vi "Stage 3.5 Placing init and close into subVIs.vi"() -> ()   [LabVIEW 2020]
uses:
  HRM-User_events.ctl
panel:
  out "Process Error":errorcluster
  out "error out":errorcluster
  out "error out Hardware":errorcluster
  in  "Addition signal to remove (0) [s]":dbl
  out "Pulse":dbl
  out "Filtered":waveform(dbl)(graph)
  in  "Samples size (10) [s]":i32=10
  out "unfiltered wf":waveform(dbl)(graph)
  in  "Stop":bool
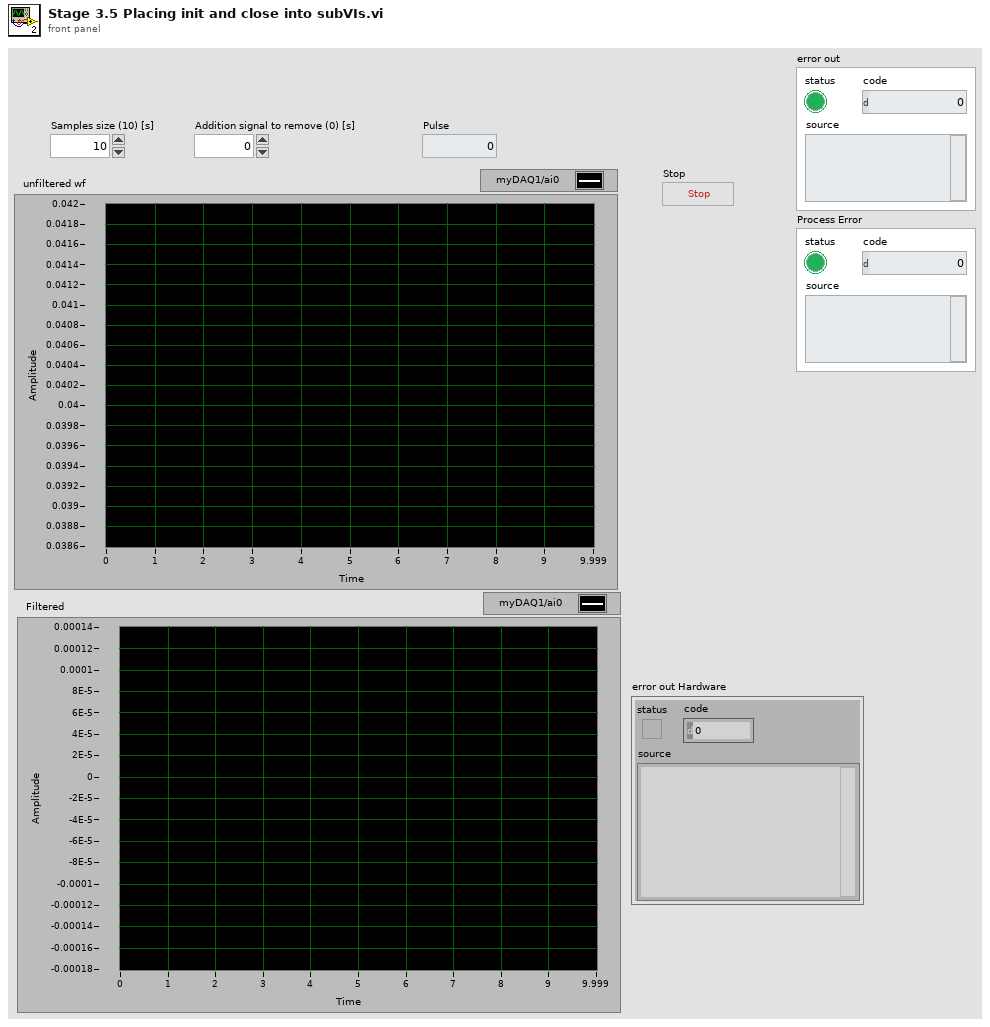
[diagram p1: front panel]
types:
  T1 = typedef "HRM-User_events.ctl" = cluster{"Signal to remove":refnum<user-event>, "Sample size":refnum<user-event>, "Filtered wf":refnum<user-event>, "Unfiltered wf":refnum<user-event>, "Raw wf":refnum<user-event>, "Pulse":refnum<user-event>, "stop":refnum<user-event>}
  T2 = typedef "HRM-init_cluster.ctl" = cluster{"User events":T1}
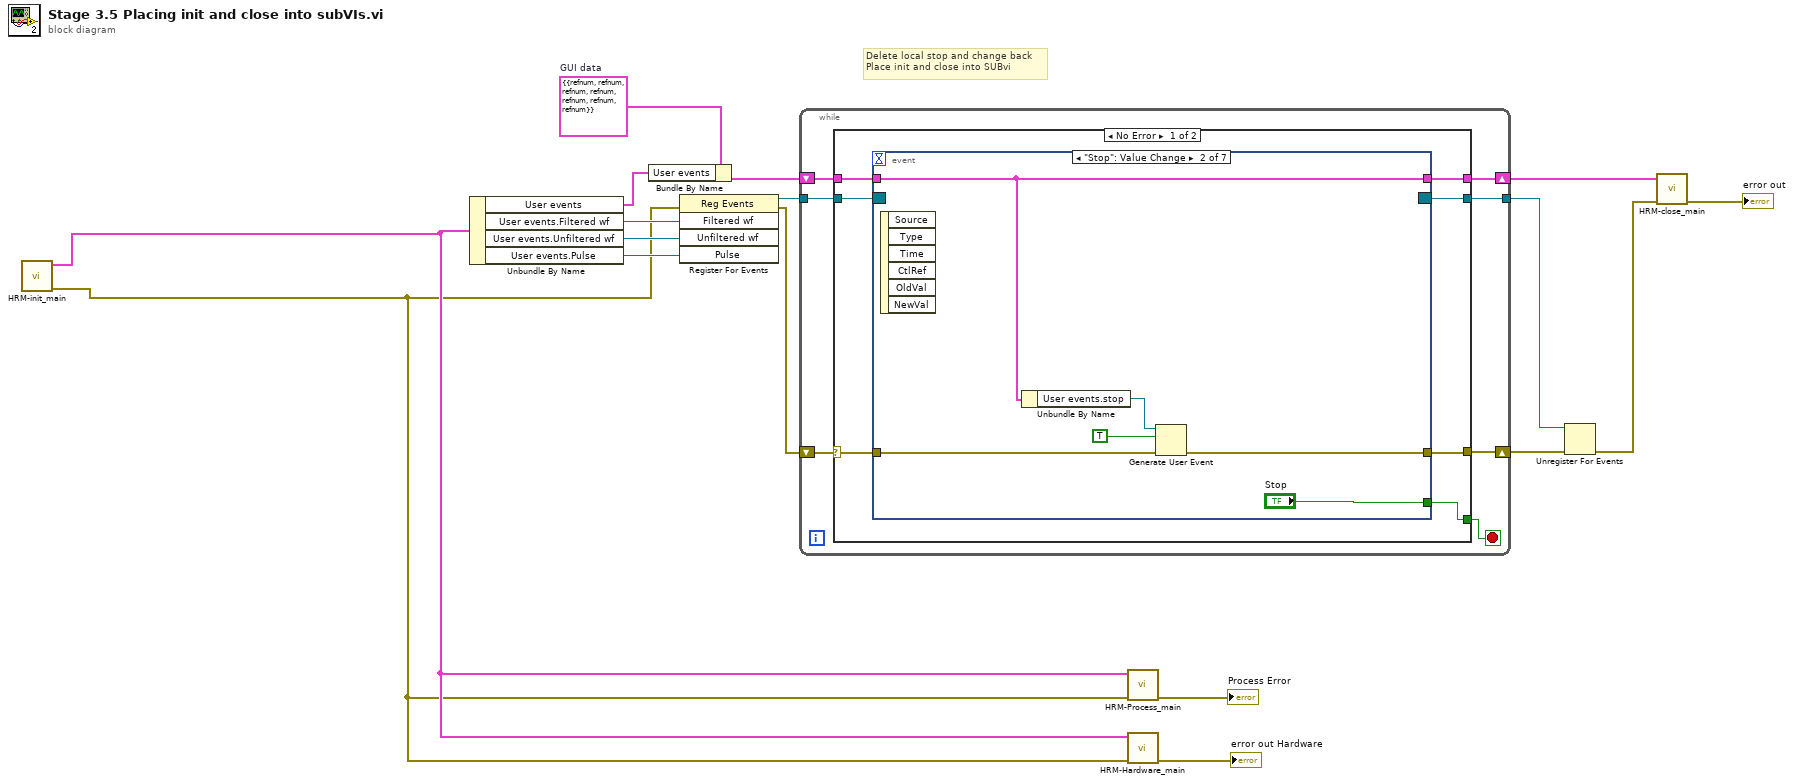
[diagram p0: block diagram]
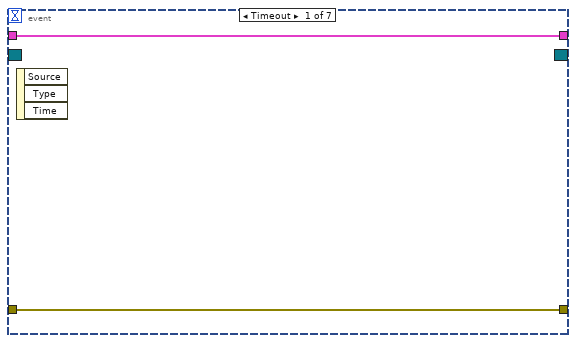
[diagram p2: hidden frame]
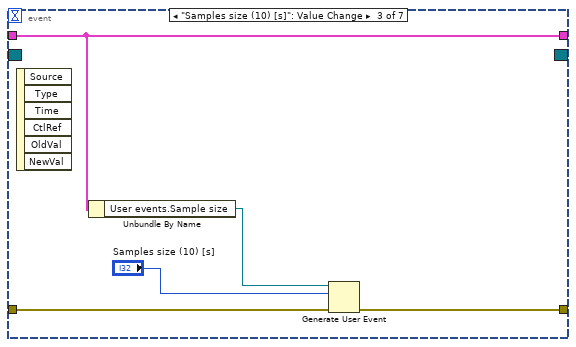
[diagram p3: hidden frame]
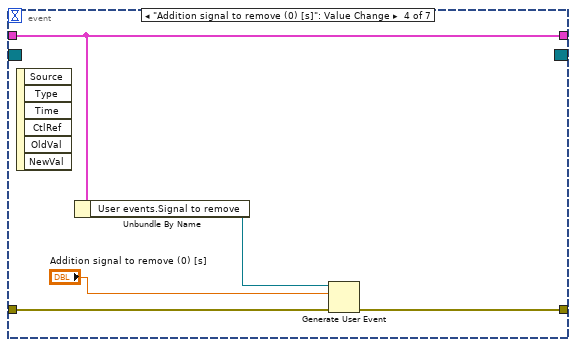
[diagram p4: hidden frame]
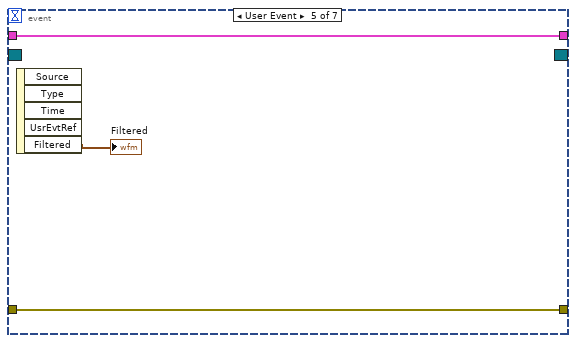
[diagram p5: hidden frame]
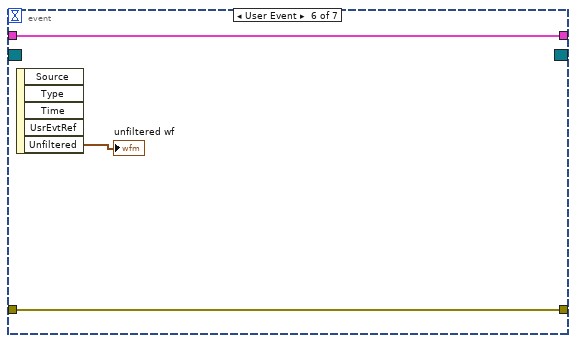
[diagram p6: hidden frame]
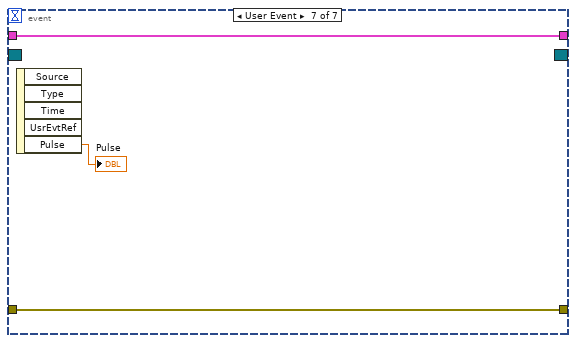
[diagram p7: hidden frame]
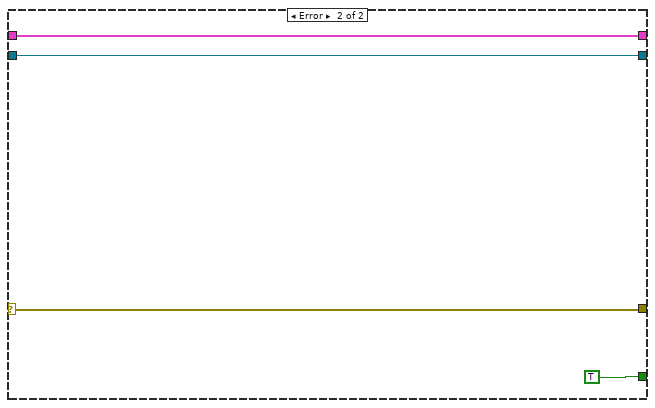
[diagram p8: hidden frame]
diagram:
  w16 = cluster{"User events":T1} {"User events"={"Signal to remove"=refnum, "Sample size"=refnum, "Filtered wf"=refnum, "Unfiltered wf"=refnum, "Raw wf"=refnum, "Pulse"=refnum, "stop"=refnum}}  # GUI data
  # "Delete local stop and change back\nPlace init and close into SUBvi"
  n1 = call "HRM-init_main.vi"() -> ("error out"=w1:errorcluster, "Init cluster"=w3:T2)  [unwired: 10 in]
  n2 = Unbundle By Name(w3) -> ("User events"=w8:T1, "User events.Filtered wf"=w7:refnum<user-event>, "User events.Unfiltered wf"=w6:refnum<user-event>, "User events.Pulse"=w5:refnum<user-event>)
  n3 = Bundle By Name(cluster=w16, "User events"=w8) -> (w9:cluster{"User events":T1})
  n4 = register-events(error in=w1, w7, w6, w5) -> (reference out=w17:refnum<event-registration>, error out=w15:errorcluster)  [unwired: 1 in]
  n5 = while {
    tunnel: w17 -> [w24]
    shift-right: [w20] -> w13
    shift-left: w15 -> [w21]
    shift-right: [w19] -> w12
    shift-left: w9 -> [w23]
    tunnel: [w18] -> w14
    stop <- w22 stop-if-true
    n6 = case shown="No Error" w21 {
      selector: w21 -> [w28 w61]
      tunnel: [w29 TRUE ("Stop")] -> w22
      tunnel: [w27 w61] -> w20
      tunnel: w24 -> [w31 w59]
      tunnel: w23 -> [w30 w60]
      tunnel: [w26 w60] -> w19
      tunnel: [w25 w59] -> w18
      frame No Error {
        n7 = event shown="[1] \"Stop\": Value Change" {
          selector: w31 -> [_ _ _ _ _ _ _]
          dyn-events: [_ _ _ _ _ _ _] -> w25
          timeout: _ -> [_ _ _ _ _ _ _]
          tunnel: w30 -> [w33 w38 w42 w47 w51 w54 w57]
          tunnel: [_ "Stop" _ _ _ _ _] -> w29
          tunnel: [w32 w35 w43 w48 w52 w55 w58] -> w27
          tunnel: w28 -> [w32 w36 w44 w49 w52 w55 w58]
          tunnel: [w33 w38 w42 w47 w51 w54 w57] -> w26
          event Timeout {
            n8 = event-data() -> ()  [unwired: 1 in, 3 out]
          }
          event "Stop": Value Change {
            n9 = event-data() -> ()  [unwired: 1 in, 6 out]
            n10 = Unbundle By Name(w38) -> ("User events.stop"=w37:refnum<user-event>)
            n11 = Generate User Event(user event=w37, event data cluster=TRUE ("event data"), error in=w36) -> (error out=w35:errorcluster)  [unwired: 1 in, 1 out]
          }
          event "Samples size (10) [s]": Value Change {
            n12 = event-data() -> ()  [unwired: 1 in, 6 out]
            n13 = Unbundle By Name(w42) -> ("User events.Sample size"=w41:refnum<user-event>)
            n14 = Generate User Event(user event=w41, event data cluster="Samples size (10) [s]", error in=w44) -> (error out=w43:errorcluster)  [unwired: 1 in, 1 out]
          }
          event "Addition signal to remove (0) [s]": Value Change {
            n15 = event-data() -> ()  [unwired: 1 in, 6 out]
            n16 = Unbundle By Name(w47) -> ("User events.Signal to remove"=w46:refnum<user-event>)
            n17 = Generate User Event(user event=w46, event data cluster="Addition signal to remove (0) [s]", error in=w49) -> (error out=w48:errorcluster)  [unwired: 1 in, 1 out]
          }
          event User Event {
            n18 = event-data() -> ("Filtered"=→"Filtered":waveform(dbl))  [unwired: 1 in, 4 out]
          }
          event User Event {
            n19 = event-data() -> ("Unfiltered"=→"unfiltered wf":waveform(dbl))  [unwired: 1 in, 4 out]
          }
          event User Event {
            n20 = event-data() -> ("Pulse"=→"Pulse":dbl)  [unwired: 1 in, 4 out]
          }
        }
      }
      frame Error {
      }
    }
  }
  n21 = call "HRM-Process_main.vi"("error in (no error)"=w1, "Init cluster"=w3) -> ("error out"=→"Process Error":errorcluster)  [unwired: 9 in]
  n22 = call "HRM-Hardware_main.vi"("error in (no error)"=w1, "Init cluster"=w3) -> ("error out"=→"error out Hardware":errorcluster)  [unwired: 9 in]
  n23 = Unregister For Events(event registration refnum=w14, error in=w13) -> (error out=w11:errorcluster)
  n24 = call "HRM-close_main.vi"("error in (no error)"=w11, "Init cluster"=w12) -> ("error out"=→"error out":errorcluster)  [unwired: 9 in]
